vi "2P_AdapUprite_Linlin.vi"() -> ()   [LabVIEW 2015] (continued)
                    n2978 = Open VI Reference(type specifier VI Refnum (for type only)=refnum<vi> refnum, vi path=w6494, error in (no error)=w6492) -> (vi reference=w6490:refnum<vi>, error out=w6488:errorcluster)  [unwired: 3 in]
                    n2979 = call-by-ref "?"(reference=w6490, error in=w6488) -> (reference out=w6489:refnum<vi>, error out=w6487:errorcluster)  [unwired: 1 in]
                    n2980 = Close Reference(reference=w6489, error in (no error)=w6487) -> (error out=w6491:errorcluster)
                    n2981 = call <vilib>:"Unset Busy.vi"("error in (no error)"=w6491) -> ()  [unwired: 10 in, 1 out]
                    n2982 = local write "status"(w6491) -> ()
                  }
                  frame #2 {
                    n2983 = call "2pparameters.vi"("command"="get") -> ("params out"=w6521:T12)  [unwired: 1 in]
                    n2984 = Unbundle By Name(w6521) -> ("Xpixels Img"=w6520:i32, "Vx-min Img"=w6519:dbl, "VX-max Img"=w6518:dbl, "Ypixels Img"=w6517:i32, "Vy-min Img"=w6516:dbl, "Vy-max Img"=w6515:dbl, "Colormap"=w6514:u16, "square pixels"=w6513:bool, "square matrix"=w6512:bool, "Angle Img"=w6511:dbl, "Drawing Mode"=w6510:u16)
                    n2985 = local write "xpixels ref"(w6520) -> ()
                    n2986 = local write "Vx-min ref"(w6519) -> ()
                    n2987 = local write "Vx-max ref"(w6518) -> ()
                    n2988 = local write "ypixels ref"(w6517) -> ()
                    n2989 = local write "Vy-min ref"(w6516) -> ()
                    n2990 = local write "Vy-max ref"(w6515) -> ()
                    n2991 = local write "Colormap"(w6514) -> ()
                    n2992 = local write "Square pixels"(w6513) -> ()
                    n2993 = local write "square matrix"(w6512) -> ()
                    n2994 = local write "Angle ref"(w6511) -> ()
                    n2995 = local write "ROI Type"(w6510) -> ()
                    n2996 = call "2pparameters.vi"("command"="get") -> ("params out"=w6504:T12)  [unwired: 1 in]
                    n2997 = Unbundle By Name(w6504) -> ("Xpixels"=w6498:i32, "Vxminref"=w6502:dbl, "Vxmaxref"=w6501:dbl, "Ypixels"=w6497:i32, "Vyminref"=w6500:dbl, "Vymaxref"=w6499:dbl, "Colormap"=w6505:u16, "square pixels"=w6506:bool, "square matrix"=w6507:bool, "Angle draw"=w6508:dbl, "Drawing Mode"=w6509:u16)
                    n2998 = local write "Vy-max draw"(w6499) -> ()
                    n2999 = local write "Angle drawing"(w6508) -> ()
                    n3000 = local write "Colormap"(w6505) -> ()
                    n3001 = local write "Square pixels"(w6506) -> ()
                    n3002 = local write "square matrix"(w6507) -> ()
                    n3003 = local write "ROI Type"(w6509) -> ()
                    n3004 = local write "xpixels draw"(w6498) -> ()
                    n3005 = local write "ypixels draw"(w6497) -> ()
                    n3006 = local write "Vx-min draw"(w6502) -> ()
                    n3007 = local write "Vx-max draw"(w6501) -> ()
                    n3008 = local write "Vy-min draw"(w6500) -> ()
                  }
                  frame #3 {
                    n3009 = property on="ROI" class="Bool (strict)"("Val(Sgnl)"=FALSE ("x/y scan")) -> ()  [unwired: 2 in, 2 out]
                  }
                }
              }
            }
          }
          event "Xdattype": Value Change {
            n3010 = event-data() -> ()  [unwired: 1 in, 1 out]
            n3011 = case shown="True" "Xdattype" {
              frame False {
              }
              frame True {
                n3012 = stacked-sequence {
                  frame #0 {
                    n3013 = Current VI's Path() -> (path=w6534:path)
                    n3014 = Strip Path(path=w6534) -> (stripped path=w6535:path)  [unwired: 1 out]
                    n3015 = Build Path(base path=w6535, name or relative path="subVIs\\Misc\\Changedataconfig.vi") -> (appended path=w6533:path)
                    n3016 = call <vilib>:"Set Busy.vi"() -> ("error out"=w6531:errorcluster)  [unwired: 10 in, 1 out]
                    n3017 = Open VI Reference(type specifier VI Refnum (for type only)=refnum<vi> refnum, vi path=w6533, error in (no error)=w6531) -> (vi reference=w6526:refnum<vi>, error out=w6528:errorcluster)  [unwired: 3 in]
                    n3018 = call-by-ref "?"(reference=w6526, error in=w6528) -> (reference out=w6530:refnum<vi>, error out=w6529:errorcluster)  [unwired: 12 in]
                    n3019 = Close Reference(reference=w6530, error in (no error)=w6529) -> (error out=w6525:errorcluster)
                    "status" <- w6525
                    n3020 = call <vilib>:"Unset Busy.vi"("error in (no error)"=w6525) -> ()  [unwired: 10 in, 1 out]
                  }
                  frame #1 {
                    n3021 = property on="Xdattype" class="Bool (strict)"("Val(Sgnl)"=FALSE ("x/y scan")) -> ()  [unwired: 2 in, 2 out]
                  }
                }
              }
            }
          }
          event "XautoOD": Value Change {
            n3022 = event-data() -> ()  [unwired: 1 in, 1 out]
            n3023 = case shown="True" "XautoOD" {
              frame False {
              }
              frame True {
                n3024 = stacked-sequence {
                  frame #0 {
                    n3025 = Current VI's Path() -> (path=w6547:path)
                    n3026 = Strip Path(path=w6547) -> (stripped path=w6548:path)  [unwired: 1 out]
                    n3027 = Build Path(base path=w6548, name or relative path="subVIs\\Misc\\ChangeautoODs.vi") -> (appended path=w6546:path)
                    n3028 = call <vilib>:"Set Busy.vi"() -> ("error out"=w6544:errorcluster)  [unwired: 10 in, 1 out]
                    n3029 = Open VI Reference(type specifier VI Refnum (for type only)=refnum<vi> refnum, vi path=w6546, error in (no error)=w6544) -> (vi reference=w6539:refnum<vi>, error out=w6541:errorcluster)  [unwired: 3 in]
                    n3030 = call-by-ref "?"(reference=w6539, error in=w6541) -> (reference out=w6543:refnum<vi>, error out=w6542:errorcluster)  [unwired: 12 in]
                    n3031 = Close Reference(reference=w6543, error in (no error)=w6542) -> (error out=w6538:errorcluster)
                    "status 2" <- w6538
                    n3032 = call <vilib>:"Unset Busy.vi"("error in (no error)"=w6538) -> ()  [unwired: 10 in, 1 out]
                  }
                  frame #1 {
                    n3033 = property on="XautoOD" class="Bool (strict)"("Val(Sgnl)"=FALSE ("x/y scan")) -> ()  [unwired: 2 in, 2 out]
                  }
                }
              }
            }
          }
          event "SetMan": Value Change {
            n3034 = event-data() -> ()  [unwired: 1 in, 1 out]
            n3035 = case shown="True" "SetMan" {
              frame False {
              }
              frame True {
                n3036 = stacked-sequence {
                  frame #0 {
                    w6551 = u16 0 items=["Rectangle", "Circle", "Freeform Boundary", "Freeform Interior"] ("ROI Type")
                    n3037 = local write "ROI Type"(w6551) -> ()
                    n3038 = local read "Square pixels"() -> (w6557:bool)
                    n3039 = case shown="False" w6557 {
                      frame False {
                        n3040 = local read "square matrix"() -> (w6558:bool)
                        n3041 = case shown="False" w6558 {
                          frame False {
                            "ypixels ref" <- "ypixels"
                            "xpixels ref" <- "xpixels"
                          }
                          frame True {
                            n3042 = local read "xpixels"() -> (w6563:i32)
                            n3043 = local read "ypixels"() -> (w6562:i32)
                            n3044 = Max & Min(x=w6563, y=w6562) -> (max(x,y)=w6561:i32)  [unwired: 1 out]
                            n3045 = local write "xpixels ref"(w6561) -> ()
                            n3046 = local write "ypixels ref"(w6561) -> ()
                          }
                        }
                      }
                      frame True {
                        n3047 = local read "square matrix"() -> (w6564:bool)
                        n3048 = case shown="True" w6564 {
                          frame False {
                            n3049 = local read "Vxmax"() -> (w6578:dbl)
                            n3050 = local read "Vx-min"() -> (w6577:dbl)
                            n3051 = local read "Vy-max"() -> (w6573:dbl)
                            n3052 = local read "Vy-min"() -> (w6574:dbl)
                            n3053 = Subtract(x=w6573, y=w6574) -> (x-y=w6575:dbl)
                            n3054 = Subtract(x=w6578, y=w6577) -> (x-y=w6576:dbl)
                            n3055 = Absolute Value(x=w6575) -> (abs(x)=w6566:dbl)
                            n3056 = Absolute Value(x=w6576) -> (abs(x)=w6567:dbl)
                            n3057 = Divide(x=w6567, y=w6566) -> (x/y=w6572:dbl)
                            n3058 = Greater Or Equal?(x=w6567, y=w6566) -> (x >= y?=w6565:bool)
                            n3059 = local read "xpixels"() -> (w6571:i32)
                            n3060 = local read "ypixels"() -> (w6568:i32)
                            n3061 = case shown="False" w6565 {
                              tunnel: w6572 -> [w6583 w6586]
                              tunnel: w6571 -> [w6580 _]
                              tunnel: [w6580 w6585] -> w6570
                              tunnel: [w6579 w6584] -> w6569
                              tunnel: w6568 -> [_ w6584]
                              frame False {
                                n3062 = To Double Precision Float(number=w6580) -> (double precision float=w6582:dbl)
                                n3063 = Divide(x=w6582, y=w6583) -> (x/y=w6581:dbl)
                                n3064 = To Long Integer(number=w6581) -> (32bit integer=w6579:i32)
                              }
                              frame True {
                                n3065 = To Double Precision Float(number=w6584) -> (double precision float=w6588:dbl)
                                n3066 = Multiply(x=w6588, y=w6586) -> (x*y=w6587:dbl)
                                n3067 = To Long Integer(number=w6587) -> (32bit integer=w6585:i32)
                              }
                            }
                            n3068 = local write "ypixels ref"(w6569) -> ()
                            n3069 = local write "xpixels ref"(w6570) -> ()
                          }
                          frame True {
                          }
                        }
                      }
                    }
                    "Vx-max ref" <- "Vxmax"
                    "Vx-min ref" <- "Vx-min"
                    "Vy-max ref" <- "Vy-max"
                    "Vy-min ref" <- "Vy-min"
                    "Angle ref" <- "Angle"
                  }
                  frame #1 {
                    n3070 = property on="SetMan" class="Bool (strict)"("Val(Sgnl)"=FALSE ("Value (Signaling)")) -> ()  [unwired: 2 in, 2 out]
                  }
                }
              }
            }
          }
          event "QuickSetMan": Value Change {
            n3071 = event-data() -> ()  [unwired: 1 in, 6 out]
            n3072 = case shown="True" "QuickSetMan" {
              tunnel: "Vpp" -> [_ w6594]
              tunnel: "px" -> [_ w6593]
              frame False {
              }
              frame True {
                n3073 = stacked-sequence {
                  tunnel: w6594 -> [w6599 _]
                  tunnel: w6593 -> [w6595 _]
                  frame #0 {
                    w6601 = u16 0 items=["Rectangle", "Circle", "Freeform Boundary", "Freeform Interior"] ("ROI Type")
                    n3074 = Divide(x=w6599, y=2.0) -> (x/y=w6598:dbl)
                    n3075 = Negate(x=w6598) -> (-x=w6597:dbl)
                    n3076 = local write "ROI Type"(w6601) -> ()
                    n3077 = local write "Vx-min ref"(w6597) -> ()
                    n3078 = local write "Vy-max ref"(w6598) -> ()
                    n3079 = local write "Vx-max ref"(w6598) -> ()
                    n3080 = local write "Vy-min ref"(w6597) -> ()
                    n3081 = local write "Angle ref"(0.0 ("Angle ref 2")) -> ()
                    n3082 = local write "xpixels ref"(w6595) -> ()
                    n3083 = local write "ypixels ref"(w6595) -> ()
                  }
                  frame #1 {
                    n3084 = property on="QuickSetMan" class="Bool (strict)"("Val(Sgnl)"=FALSE ("Value (Signaling)")) -> ()  [unwired: 2 in, 2 out]
                  }
                }
              }
            }
          }
          event "SetMan 2": Value Change {
            n3085 = event-data() -> ()  [unwired: 1 in, 1 out]
            n3086 = case shown="True" "SetMan 2" {
              frame False {
              }
              frame True {
                n3087 = stacked-sequence {
                  frame #0 {
                    n3088 = local write "Vx-ref"("Vx") -> ()
                    n3089 = local write "Vy-ref"("Vy") -> ()
                  }
                  frame #1 {
                    n3090 = property on="SetMan 2" class="Bool (strict)"("Val(Sgnl)"=FALSE ("Value (Signaling)")) -> ()  [unwired: 2 in, 2 out]
                  }
                }
              }
            }
          }
          event "Reset Coords": Value Change {
            n3091 = event-data() -> ("NewVal"=w6607:bool)  [unwired: 1 in, 5 out]
            n3092 = case shown="True" w6607 {
              frame False {
              }
              frame True {
                n3093 = stacked-sequence {
                  frame #0 {
                    n3094 = local write "xpixels"(256 ("xpixels")) -> ()
                    n3095 = local write "ypixels"(256 ("ypixels")) -> ()
                    n3096 = local write "Vxmax"(9.0 ("Vx-max")) -> ()
                    n3097 = local write "Vx-min"(-9.0 ("Vx-min")) -> ()
                    n3098 = local write "Vy-max"(9.0 ("Vy-max")) -> ()
                    n3099 = local write "Vy-min"(-9.0 ("Vy-min")) -> ()
                    n3100 = local write "Angle"(0.0 ("Angle")) -> ()
                  }
                  frame #1 {
                    n3101 = property on="Reset Coords" class="Bool (strict)"("Value"=FALSE ("TROI")) -> ()  [unwired: 2 in, 2 out]
                  }
                }
              }
            }
          }
          event "TROI": Value Change {
            n3102 = event-data() -> ()  [unwired: 1 in, 1 out]
            n3103 = case shown="True" "TROI" {
              frame False {
              }
              frame True {
                n3104 = stacked-sequence {
                  frame #0 {
                    n3105 = local read "Vy-min ref"() -> (w6621:dbl)
                    n3106 = local read "Vy-max ref"() -> (w6620:dbl)
                    n3107 = local read "Vx-max ref"() -> (w6618:dbl)
                    n3108 = local read "Vx-min ref"() -> (w6619:dbl)
                    n3109 = local read "ypixels ref"() -> (w6623:i32)
                    n3110 = local read "xpixels ref"() -> (w6622:i32)
                    n3111 = local read "Angle ref"() -> (w6617:dbl)
                    n3112 = local write "Angle"(w6617) -> ()
                    n3113 = local write "xpixels"(w6622) -> ()
                    n3114 = local write "Vy-min"(w6621) -> ()
                    n3115 = local write "Vy-max"(w6620) -> ()
                    n3116 = local write "Vx-min"(w6619) -> ()
                    n3117 = local write "ypixels"(w6623) -> ()
                    n3118 = local write "Vxmax"(w6618) -> ()
                  }
                  frame #1 {
                    n3119 = property on="TROI" class="Bool (strict)"("Value"=FALSE ("TROI")) -> ()  [unwired: 2 in, 2 out]
                  }
                }
              }
            }
          }
          event "TROI 2": Value Change {
            n3120 = event-data() -> ()  [unwired: 1 in, 1 out]
            n3121 = case shown="True" "TROI 2" {
              frame False {
              }
              frame True {
                n3122 = stacked-sequence {
                  frame #0 {
                    n3123 = local read "Vx-ref"() -> (w6626:dbl)
                    n3124 = local read "Vy-ref"() -> (w6627:dbl)
                    n3125 = local write "Vx"(w6626) -> ()
                    n3126 = local write "Vy"(w6627) -> ()
                  }
                  frame #1 {
                    n3127 = property on="TROI 2" class="Bool (strict)"("Value"=FALSE ("TROI")) -> ()  [unwired: 2 in, 2 out]
                  }
                }
              }
            }
          }
          event "Square pixels": Value Change {
            n3128 = event-data() -> ()  [unwired: 1 in, 1 out]
            n3129 = case shown="True" "Square pixels" {
              frame False {
              }
              frame True {
                n3130 = property on="square matrix" class="Bool (strict)"("Value"=FALSE ("square matrix")) -> ()  [unwired: 2 in, 2 out]
                n3131 = property on="Square pixels" class="Bool (strict)"("Value"=TRUE ("square matrix")) -> ()  [unwired: 2 in, 2 out]
              }
            }
          }
          event "square matrix": Value Change {
            n3132 = event-data() -> ()  [unwired: 1 in, 1 out]
            n3133 = case shown="True" "square matrix" {
              frame False {
              }
              frame True {
                n3134 = property on="square matrix" class="Bool (strict)"("Value"=TRUE ("square matrix")) -> ()  [unwired: 2 in, 2 out]
                n3135 = property on="Square pixels" class="Bool (strict)"("Value"=FALSE ("square matrix")) -> ()  [unwired: 2 in, 2 out]
              }
            }
          }
          event "up", "downright", "down", "downleft", "right", "left", "upright", "upleft": Value Change {
            n3136 = event-data() -> ()  [unwired: 1 in, 6 out]
            n3137 = local read "downright"() -> (w6640:bool)
            n3138 = local read "downleft"() -> (w6642:bool)
            n3139 = local read "upright"() -> (w6638:bool)
            n3140 = local read "upleft"() -> (w6636:bool)
            n3141 = local read "down"() -> (w6641:bool)
            n3142 = local read "right"() -> (w6639:bool)
            n3143 = local read "left"() -> (w6643:bool)
            n3144 = local read "up"() -> (w6637:bool)
            n3145 = Compound Arithmetic op=OR(w6636, w6637, w6638, w6639, w6640, w6641, w6642, w6643) -> (w6635:bool)
            n3146 = case shown="True" w6635 {
              frame False {
              }
              frame True {
                n3147 = stacked-sequence {
                  frame #0 {
                    n3148 = local read "downright"() -> (w6645:bool)
                    n3149 = local read "downleft"() -> (w6647:bool)
                    n3150 = local read "BigSmall"() -> (w6644:bool)
                    n3151 = local read "upright"() -> (w6649:bool)
                    n3152 = local read "upleft"() -> (w6652:bool)
                    n3153 = local read "down"() -> (w6648:bool)
                    n3154 = local read "right"() -> (w6650:bool)
                    n3155 = local read "left"() -> (w6646:bool)
                    n3156 = local read "up"() -> (w6651:bool)
                    n3157 = call "movestageparams.vi"("command"="get") -> ("Params out"=w6655:T23)  [unwired: 1 in]
                    n3158 = Bundle By Name(cluster=w6655, "upleft"=w6652, "up"=w6651, "upright"=w6649, "right"=w6650, "downright"=w6645, "down"=w6648, "downleft"=w6647, "left"=w6646, "Bigsmall"=w6644) -> (w6656:T23)
                    n3159 = call "movestageparams.vi"("Params in"=w6656, "command"="set") -> ()  [unwired: 1 out]
                  }
                  frame #1 {
                  }
                  frame #2 {
                    n3160 = call "movestage.vi"() -> ()  [unwired: 12 in]
                  }
                  frame #3 {
                    w6657 = FALSE ("OK Button")
                    w6658 = FALSE ("OK Button")
                    n3161 = property on="down" class="Bool (strict)"("Value"=w6658) -> ()  [unwired: 2 in, 2 out]
                    n3162 = property on="up" class="Bool (strict)"("Value"=w6658) -> ()  [unwired: 2 in, 2 out]
                    n3163 = property on="right" class="Bool (strict)"("Value"=w6658) -> ()  [unwired: 2 in, 2 out]
                    n3164 = property on="left" class="Bool (strict)"("Value"=w6658) -> ()  [unwired: 2 in, 2 out]
                    n3165 = property on="upright" class="Bool (strict)"("Value"=w6657) -> ()  [unwired: 2 in, 2 out]
                    n3166 = property on="downleft" class="Bool (strict)"("Value"=w6657) -> ()  [unwired: 2 in, 2 out]
                    n3167 = property on="downright" class="Bool (strict)"("Value"=w6657) -> ()  [unwired: 2 in, 2 out]
                    n3168 = property on="upleft" class="Bool (strict)"("Value"=w6657) -> ()  [unwired: 2 in, 2 out]
                  }
                }
              }
            }
          }
          event "finite samples": Value Change {
            n3169 = event-data() -> ("NewVal"=w6659:bool)  [unwired: 1 in]
            n3170 = flat-sequence {
              tunnel: w6659 -> [w6660]
              frame #0 {
                n3171 = case shown="True" w6660 {
                  frame False {
                    w6661 = FALSE ("wavdet")
                    n3172 = property on="continuous" class="Bool (strict)"("Value"=TRUE ("continuous for display")) -> ()  [unwired: 2 in, 2 out]
                    n3173 = property on="wavdet" class="Bool (strict)"("Value"=w6661) -> ()  [unwired: 2 in, 2 out]
                    n3174 = property on="save\ndata" class="Bool (strict)"("Value"=w6661) -> ()  [unwired: 2 in, 2 out]
                    n3175 = property on="# of frames" class="DigNum (strict)"("DisabledEnum"=T7."Disabled and Grayed Out" ("Disabled")) -> ()  [unwired: 2 in, 2 out]
                    n3176 = property on="save\ndata" class="Bool (strict)"("DisabledEnum"=T7."Disabled and Grayed Out" ("Disabled")) -> ()  [unwired: 2 in, 2 out]
                    "Save tab" <- enum32{"withsave", "withoutsave"}."withsave" ("Save tab")
                  }
                  frame True {
                    w6668 = FALSE ("continuous for display")
                    n3177 = property on="continuous" class="Bool (strict)"("Value"=w6668) -> ()  [unwired: 2 in, 2 out]
                    n3178 = property on="wavdet" class="Bool (strict)"("Value"=w6668) -> ()  [unwired: 2 in, 2 out]
                    n3179 = local write "Save tab"(enum32{"withsave", "withoutsave"}."withsave" ("Save tab")) -> ()
                    n3180 = property on="save\ndata" class="Bool (strict)"("DisabledEnum"=T7."Enabled" ("Disabled")) -> ()  [unwired: 2 in, 2 out]
                    n3181 = property on="save\ndata" class="Bool (strict)"("Value"=TRUE ("save\ndata")) -> ()  [unwired: 2 in, 2 out]
                    n3182 = property on="# of frames" class="DigNum (strict)"("DisabledEnum"=T7."Enabled" ("Disabled")) -> ()  [unwired: 2 in, 2 out]
                  }
                }
              }
              frame #1 {
                n3183 = local read "finite samples"() -> (w6677:bool)
                n3184 = local read "continuous"() -> (w6676:bool)
                n3185 = local read "wavdet"() -> (w6675:bool)
                n3186 = call "2pparameters.vi"("command"="get") -> ("params out"=w6671:T12)  [unwired: 1 in]
                n3187 = Bundle By Name(cluster=w6671, "finite"=w6677, "cont"=w6676, "wavdet"=w6675) -> (w6674:T12)
                n3188 = call "2pparameters.vi"("Params in"=w6674, "command"="set") -> ()  [unwired: 1 out]
              }
            }
          }
          event "continuous": Value Change {
            n3189 = event-data() -> ("NewVal"=w6678:bool)  [unwired: 1 in]
            n3190 = flat-sequence {
              tunnel: w6678 -> [w6679]
              frame #0 {
                n3191 = case shown="True" w6679 {
                  frame False {
                    n3192 = property on="finite samples" class="Bool (strict)"("Value"=TRUE ("finite samples for recording")) -> ()  [unwired: 2 in, 2 out]
                    n3193 = property on="save\ndata" class="Bool (strict)"("Value"=TRUE ("save\ndata")) -> ()  [unwired: 2 in, 2 out]
                    n3194 = property on="wavdet" class="Bool (strict)"("Value"=FALSE ("wavdet")) -> ()  [unwired: 2 in, 2 out]
                    n3195 = local write "Save tab"(enum32{"withsave", "withoutsave"}."withsave" ("Save tab")) -> ()
                    n3196 = property on="# of frames" class="DigNum (strict)"("DisabledEnum"=T7."Enabled" ("Disabled")) -> ()  [unwired: 2 in, 2 out]
                    n3197 = property on="save\ndata" class="Bool (strict)"("DisabledEnum"=T7."Enabled" ("Disabled")) -> ()  [unwired: 2 in, 2 out]
                  }
                  frame True {
                    w6686 = FALSE ("finite samples for recording")
                    n3198 = property on="finite samples" class="Bool (strict)"("Value"=w6686) -> ()  [unwired: 2 in, 2 out]
                    n3199 = property on="wavdet" class="Bool (strict)"("Value"=w6686) -> ()  [unwired: 2 in, 2 out]
                    n3200 = property on="save\ndata" class="Bool (strict)"("Value"=w6686) -> ()  [unwired: 2 in, 2 out]
                    n3201 = local write "Save tab"(enum32{"withsave", "withoutsave"}."withsave" ("Save tab")) -> ()
                    n3202 = property on="# of frames" class="DigNum (strict)"("DisabledEnum"=T7."Disabled and Grayed Out" ("Disabled")) -> ()  [unwired: 2 in, 2 out]
                    n3203 = property on="save\ndata" class="Bool (strict)"("DisabledEnum"=T7."Disabled and Grayed Out" ("Disabled")) -> ()  [unwired: 2 in, 2 out]
                  }
                }
              }
              frame #1 {
                n3204 = local read "finite samples"() -> (w6696:bool)
                n3205 = local read "continuous"() -> (w6695:bool)
                n3206 = local read "wavdet"() -> (w6694:bool)
                n3207 = call "2pparameters.vi"("command"="get") -> ("params out"=w6690:T12)  [unwired: 1 in]
                n3208 = Bundle By Name(cluster=w6690, "finite"=w6696, "cont"=w6695, "wavdet"=w6694) -> (w6693:T12)
                n3209 = call "2pparameters.vi"("Params in"=w6693, "command"="set") -> ()  [unwired: 1 out]
              }
            }
          }
          event "wavdet": Value Change {
            n3210 = event-data() -> ("NewVal"=w6697:bool)  [unwired: 1 in]
            n3211 = flat-sequence {
              tunnel: w6697 -> [w6698]
              frame #0 {
                n3212 = case shown="False" w6698 {
                  frame False {
                    n3213 = property on="finite samples" class="Bool (strict)"("Value"=TRUE ("finite samples for recording")) -> ()  [unwired: 2 in, 2 out]
                    n3214 = property on="continuous" class="Bool (strict)"("Value"=FALSE ("continuous")) -> ()  [unwired: 2 in, 2 out]
                    n3215 = local write "Save tab"(enum32{"withsave", "withoutsave"}."withsave" ("Save tab")) -> ()
                    n3216 = property on="save\ndata" class="Bool (strict)"("DisabledEnum"=T7."Enabled" ("Disabled")) -> ()  [unwired: 2 in, 2 out]
                    n3217 = property on="# of frames" class="DigNum (strict)"("DisabledEnum"=T7."Enabled" ("Disabled")) -> ()  [unwired: 2 in, 2 out]
                    n3218 = property on="save\ndata" class="Bool (strict)"("Value"=TRUE ("save\ndata")) -> ()  [unwired: 2 in, 2 out]
                  }
                  frame True {
                    w6707 = FALSE ("finite samples for recording")
                    n3219 = property on="finite samples" class="Bool (strict)"("Value"=w6707) -> ()  [unwired: 2 in, 2 out]
                    n3220 = property on="continuous" class="Bool (strict)"("Value"=w6707) -> ()  [unwired: 2 in, 2 out]
                    n3221 = property on="save\ndata" class="Bool (strict)"("DisabledEnum"=T7."Enabled" ("Disabled")) -> ()  [unwired: 2 in, 2 out]
                    n3222 = local write "Save tab"(enum32{"withsave", "withoutsave"}."withsave" ("Save tab")) -> ()
                    n3223 = property on="# of frames" class="DigNum (strict)"("DisabledEnum"=T7."Disabled" ("Disabled")) -> ()  [unwired: 2 in, 2 out]
                    n3224 = property on="save\ndata" class="Bool (strict)"("Value"=TRUE ("save\ndata")) -> ()  [unwired: 2 in, 2 out]
                  }
                }
              }
              frame #1 {
                n3225 = local read "finite samples"() -> (w6710:bool)
                n3226 = local read "continuous"() -> (w6711:bool)
                n3227 = local read "wavdet"() -> (w6712:bool)
                n3228 = call "2pparameters.vi"("command"="get") -> ("params out"=w6716:T12)  [unwired: 1 in]
                n3229 = Bundle By Name(cluster=w6716, "finite"=w6710, "cont"=w6711, "wavdet"=w6712) -> (w6713:T12)
                n3230 = call "2pparameters.vi"("Params in"=w6713, "command"="set") -> ()  [unwired: 1 out]
              }
            }
          }
          event "cursors": Value Change {
            n3231 = event-data() -> ()  [unwired: 1 in, 5 out]
            n3232 = case shown="True" "cursors" {
              frame False {
                n3233 = property on="img_CH1" class="IntGraph (strict)"("Active Cursor"=u32 0, "Cursor.Cursor Style"=u8 0 ("Cursor Style"), "Cursor.Cursor Point Style"=u8 0 ("Cursor Point Style")) -> ("Cursor.Cursor Position:Cursor X"=w6721:dbl, "Cursor.Cursor Position:Cursor Y"=w6722:dbl)  [unwired: 2 in, 2 out]
                n3234 = property on="img_CH2" class="IntGraph (strict)"("Active Cursor"=u32 0, "Cursor.Cursor Style"=u8 0 ("Cursor Style"), "Cursor.Cursor Point Style"=u8 0 ("Cursor Point Style")) -> ()  [unwired: 2 in, 2 out]
                n3235 = local write "cursor x [pixel]"(w6721) -> ()
                n3236 = local write "cursor y [pixel]"(w6722) -> ()
              }
              frame True {
                n3237 = stacked-sequence {
                  frame #0 {
                    n3238 = call "2pparameters.vi"("command"="get") -> ("params out"=w6737:T12)  [unwired: 1 in]
                    n3239 = Unbundle By Name(w6737) -> ("Xpixels Img"=w6738:i32, "Ypixels Img"=w6735:i32)
                    n3240 = To Double Precision Float(number=w6735) -> (double precision float=w6729:dbl)
                    n3241 = To Double Precision Float(number=w6738) -> (double precision float=w6734:dbl)
                    n3242 = Divide(x=w6729, y=2.0) -> (x/y=w6730:dbl)
                    n3243 = Divide(x=w6734, y=2.0) -> (x/y=w6732:dbl)
                    n3244 = Round To Nearest(number=w6730) -> (nearest integer value=w6728:dbl)
                    n3245 = Round To Nearest(number=w6732) -> (nearest integer value=w6731:dbl)
                    n3246 = property on="img_CH1" class="IntGraph (strict)"("Active Cursor"=u32 0, "Cursor.Cursor Style"=u8 8 ("Cursor Style"), "Cursor.Cursor Point Style"=u8 5 ("Cursor Point Style"), "Cursor.Cursor Position:Cursor X"=w6731, "Cursor.Cursor Position:Cursor Y"=w6728, "Cursor.Visible"=TRUE) -> ()  [unwired: 2 in, 2 out]
                  }
                  frame #1 {
                    n3247 = call "2pparameters.vi"("command"="get") -> ("params out"=w6757:T12)  [unwired: 1 in]
                    n3248 = call "2pparameters.vi"("command"="get") -> ("params out"=w6755:T12)  [unwired: 1 in]
                    n3249 = property on="img_CH1" class="IntGraph (strict)"("Active Cursor"=u32 0, "Cursor.Cursor Style"=u8 8 ("Cursor Style"), "Cursor.Cursor Point Style"=u8 5 ("Cursor Point Style")) -> ("Cursor.Cursor Position:Cursor X"=w6750:dbl, "Cursor.Cursor Position:Cursor Y"=w6749:dbl, "Cursor.Cursor Index"=w6772:i32, "Cursor.Cursor Plot"=w6771:i32, "Cursor.Visible"=w6742:bool)  [unwired: 2 in, 2 out]
                    "cursor x [pixel]" <- w6750
                    "cursor y [pixel]" <- w6749
                    n3250 = Unbundle By Name(w6757) -> ("Vy-max Img"=w6759:dbl, "Vy-min Img"=w6746:dbl, "Ypixels Img"=w6761:i32)
                    n3251 = Unbundle By Name(w6755) -> ("VX-max Img"=w6756:dbl, "Vx-min Img"=w6744:dbl, "Xpixels Img"=w6760:i32)
                    n3252 = Subtract(x=w6759, y=w6746) -> (x-y=w6764:dbl)
                    n3253 = Subtract(x=w6756, y=w6744) -> (x-y=w6762:dbl)
                    n3254 = local read "img_CH2"() -> (w6768:sgl[][])
                    n3255 = To Double Precision Float(number=w6760) -> (double precision float=w6763:dbl)
                    n3256 = local read "img_CH1"() -> (w6769:sgl[][])
                    n3257 = To Double Precision Float(number=w6761) -> (double precision float=w6765:dbl)
                    n3258 = Index Array(array=w6769, index (row)=w6772, index (col)=w6771) -> (element=→"value CH 1":sgl)
                    n3259 = Index Array(array=w6768, index (row)=w6772, index (col)=w6771) -> (element=→"value CH 2":sgl)
                    n3260 = Divide(x=w6762, y=w6763) -> (x/y=w6766:dbl)
                    n3261 = Divide(x=w6764, y=w6765) -> (x/y=w6767:dbl)
                    n3262 = Multiply(x=w6750, y=w6766) -> (x*y=w6745:dbl)
                    n3263 = Multiply(x=w6749, y=w6767) -> (x*y=w6748:dbl)
                    n3264 = property on="img_CH2" class="IntGraph (strict)"("Active Cursor"=u32 0, "Cursor.Cursor Style"=u8 8 ("Cursor Style"), "Cursor.Cursor Point Style"=u8 5 ("Cursor Point Style"), "Cursor.Cursor Position:Cursor X"=w6750, "Cursor.Cursor Position:Cursor Y"=w6749, "Cursor.Visible"=w6742) -> ()  [unwired: 2 in, 2 out]
                    n3265 = Add(x=w6745, y=w6744) -> (x+y=w6743:dbl)
                    n3266 = Add(x=w6748, y=w6746) -> (x+y=w6747:dbl)
                    n3267 = local write "Vx-ref"(w6743) -> ()
                    n3268 = local write "Vy-ref"(w6747) -> ()
                  }
                }
              }
            }
          }
          event "img_CH1": Cursor Move {
            n3269 = event-data() -> ("CursIdx"=w6777:i32)  [unwired: 1 in]
            n3270 = Equal To 0?(x=w6777) -> (x = 0?=w6778:bool)
            n3271 = case shown="True" w6778 {
              frame False {
              }
              frame True {
                n3272 = call "2pparameters.vi"("command"="get") -> ("params out"=w6798:T12)  [unwired: 1 in]
                n3273 = call "2pparameters.vi"("command"="get") -> ("params out"=w6800:T12)  [unwired: 1 in]
                n3274 = property on="img_CH1" class="IntGraph (strict)"("Active Cursor"=u32 0, "Cursor.Cursor Style"=u8 8 ("Cursor Style"), "Cursor.Cursor Point Style"=u8 5 ("Cursor Point Style")) -> ("Cursor.Cursor Position:Cursor X"=w6787:dbl, "Cursor.Cursor Position:Cursor Y"=w6786:dbl, "Cursor.Cursor Plot"=w6806:i32, "Cursor.Cursor Index"=w6805:i32, "Cursor.Visible"=w6779:bool)  [unwired: 2 in, 2 out]
                n3275 = Unbundle By Name(w6798) -> ("Vy-max Img"=w6796:dbl, "Vy-min Img"=w6785:dbl, "Ypixels Img"=w6794:i32)
                n3276 = Unbundle By Name(w6800) -> ("VX-max Img"=w6799:dbl, "Vx-min Img"=w6780:dbl, "Xpixels Img"=w6795:i32)
                n3277 = Subtract(x=w6796, y=w6785) -> (x-y=w6791:dbl)
                n3278 = Subtract(x=w6799, y=w6780) -> (x-y=w6793:dbl)
                n3279 = local write "cursor x [pixel]"(w6787) -> ()
                n3280 = local write "cursor y [pixel]"(w6786) -> ()
                n3281 = To Double Precision Float(number=w6795) -> (double precision float=w6792:dbl)
                n3282 = To Double Precision Float(number=w6794) -> (double precision float=w6790:dbl)
                n3283 = local read "img_CH2"() -> (w6807:sgl[][])
                n3284 = local read "img_CH1"() -> (w6810:sgl[][])
                n3285 = Index Array(array=w6807, index (row)=w6806, index (col)=w6805) -> (element=w6808:sgl)
                n3286 = Index Array(array=w6810, index (row)=w6806, index (col)=w6805) -> (element=w6809:sgl)
                n3287 = Divide(x=w6793, y=w6792) -> (x/y=w6789:dbl)
                n3288 = Divide(x=w6791, y=w6790) -> (x/y=w6788:dbl)
                n3289 = local write "value CH 2"(w6808) -> ()
                n3290 = Multiply(x=w6787, y=w6789) -> (x*y=w6782:dbl)
                n3291 = local write "value CH 1"(w6809) -> ()
                n3292 = Multiply(x=w6786, y=w6788) -> (x*y=w6784:dbl)
                n3293 = Add(x=w6782, y=w6780) -> (x+y=w6781:dbl)
                n3294 = local write "Vx-ref"(w6781) -> ()
                n3295 = Add(x=w6784, y=w6785) -> (x+y=w6783:dbl)
                n3296 = property on="img_CH2" class="IntGraph (strict)"("Active Cursor"=u32 0, "Cursor.Cursor Style"=u8 8 ("Cursor Style"), "Cursor.Cursor Point Style"=u8 5 ("Cursor Point Style"), "Cursor.Cursor Position:Cursor X"=w6787, "Cursor.Cursor Position:Cursor Y"=w6786, "Cursor.Visible"=w6779) -> ()  [unwired: 2 in, 2 out]
                n3297 = local write "Vy-ref"(w6783) -> ()
              }
            }
          }
          event "img_CH2": Cursor Move {
            n3298 = event-data() -> ("CursIdx"=w6814:i32)  [unwired: 1 in]
            n3299 = Equal To 0?(x=w6814) -> (x = 0?=w6815:bool)
            n3300 = case shown="True" w6815 {
              frame False {
              }
              frame True {
                n3301 = property on="img_CH2" class="IntGraph (strict)"("Active Cursor"=u32 0, "Cursor.Cursor Style"=u8 8 ("Cursor Style"), "Cursor.Cursor Point Style"=u8 5 ("Cursor Point Style")) -> ("Cursor.Cursor Position:Cursor X"=w6823:dbl, "Cursor.Cursor Position:Cursor Y"=w6824:dbl, "Cursor.Cursor Plot"=w6843:i32, "Cursor.Cursor Index"=w6842:i32, "Cursor.Visible"=w6816:bool)  [unwired: 2 in, 2 out]
                n3302 = call "2pparameters.vi"("command"="get") -> ("params out"=w6835:T12)  [unwired: 1 in]
                n3303 = call "2pparameters.vi"("command"="get") -> ("params out"=w6837:T12)  [unwired: 1 in]
                n3304 = local read "img_CH1"() -> (w6847:sgl[][])
                n3305 = local read "img_CH2"() -> (w6844:sgl[][])
                n3306 = local write "cursor x [pixel]"(w6823) -> ()
                n3307 = local write "cursor y [pixel]"(w6824) -> ()
                n3308 = Unbundle By Name(w6835) -> ("Vy-max Img"=w6833:dbl, "Vy-min Img"=w6818:dbl, "Ypixels Img"=w6831:i32)
                n3309 = Unbundle By Name(w6837) -> ("VX-max Img"=w6836:dbl, "Vx-min Img"=w6821:dbl, "Xpixels Img"=w6832:i32)
                n3310 = Index Array(array=w6847, index (row)=w6843, index (col)=w6842) -> (element=w6846:sgl)
                n3311 = Index Array(array=w6844, index (row)=w6843, index (col)=w6842) -> (element=w6845:sgl)
                n3312 = local write "value CH 2"(w6845) -> ()
                n3313 = local write "value CH 1"(w6846) -> ()
                n3314 = Subtract(x=w6833, y=w6818) -> (x-y=w6828:dbl)
                n3315 = Subtract(x=w6836, y=w6821) -> (x-y=w6830:dbl)
                n3316 = To Double Precision Float(number=w6832) -> (double precision float=w6829:dbl)
                n3317 = To Double Precision Float(number=w6831) -> (double precision float=w6827:dbl)
                n3318 = Divide(x=w6830, y=w6829) -> (x/y=w6826:dbl)
                n3319 = Divide(x=w6828, y=w6827) -> (x/y=w6825:dbl)
                n3320 = Multiply(x=w6823, y=w6826) -> (x*y=w6822:dbl)
                n3321 = Multiply(x=w6824, y=w6825) -> (x*y=w6819:dbl)
                n3322 = property on="img_CH1" class="IntGraph (strict)"("Active Cursor"=u32 0, "Cursor.Cursor Style"=u8 8 ("Cursor Style"), "Cursor.Cursor Point Style"=u8 5 ("Cursor Point Style"), "Cursor.Cursor Position:Cursor X"=w6823, "Cursor.Cursor Position:Cursor Y"=w6824, "Cursor.Visible"=w6816) -> ()  [unwired: 2 in, 2 out]
                n3323 = Add(x=w6822, y=w6821) -> (x+y=→"Vx-ref":dbl)
                n3324 = Add(x=w6819, y=w6818) -> (x+y=→"Vy-ref":dbl)
              }
            }
          }
          event "Focus": Value Change {
            n3325 = event-data() -> ()  [unwired: 1 in, 6 out]
            n3326 = flat-sequence {
              frame #0 {
                n3327 = local read "Focus"() -> (w6851:bool)
                n3328 = case shown="True" w6851 {
                  frame False {
                  }
                  frame True {
                    n3329 = local read "Vx-ref"() -> (w6855:dbl)
                    n3330 = local read "Vy-ref"() -> (w6854:dbl)
                    n3331 = local read "zV"() -> (w6852:dbl)
                    n3332 = call "focusvi.vi"("zc"=w6852, "yc"=w6854, "xc"=w6855) -> ("finalz"=→"zV":dbl)
                  }
                }
              }
              frame #1 {
                n3333 = local write "Focus"(FALSE ("Focus")) -> ()
              }
            }
          }
          event "auto shutter": Value Change {
            n3334 = event-data() -> ()  [unwired: 1 in, 6 out]
            n3335 = call "2pparameters.vi"("command"="get") -> ("params out"=w6859:T12)  [unwired: 1 in]
            n3336 = in-place {
              n3337 = in-place-cluster #45(w6859) -> ()  [unwired: 1 out]
              n3338 = local read "auto shutter"() -> (w6861:bool)
              n3339 = in-place-cluster #45("autoshutter"=w6861) -> (w6857:T12)
            }
            n3340 = call "2pparameters.vi"("Params in"=w6857, "command"="set") -> ()  [unwired: 1 out]
          }
          event "auto OD": Value Change {
            n3341 = event-data() -> ()  [unwired: 1 in, 6 out]
            n3342 = call "2pparameters.vi"("command"="get") -> ("params out"=w6864:T12)  [unwired: 1 in]
            n3343 = in-place {
              n3344 = in-place-cluster #46(w6864) -> ()  [unwired: 1 out]
              n3345 = local read "auto OD"() -> (w6866:bool)
              n3346 = in-place-cluster #46("auto OD"=w6866) -> (w6862:T12)
            }
            n3347 = call "2pparameters.vi"("Params in"=w6862, "command"="set") -> ()  [unwired: 1 out]
          }
          event "ODfilt": Value Change {
            n3348 = event-data() -> ("OldVal"=w6869:u16)  [unwired: 1 in, 5 out]
            n3349 = call "2pparameters.vi"("command"="get") -> ("params out"=w6867:T12)  [unwired: 1 in]
            n3350 = local read "ODfilt"() -> (w6870:u16)
            n3351 = call "filterwheelcontrol_nothorlabslib.vi"("Current OD filt"=w6869, "New ODfilt"=w6870) -> ()  [unwired: 1 in]
            n3352 = in-place {
              in-place-border: w6870 -> [w6873]
              n3353 = in-place-cluster #47(w6867) -> ()  [unwired: 1 out]
              n3354 = in-place-cluster #47("ODfilt"=w6873) -> (w6871:T12)
            }
            n3355 = call "2pparameters.vi"("Params in"=w6871, "command"="set") -> ()  [unwired: 1 out]
          }
          event "Use external 100KHz Clock": Value Change {
            n3356 = event-data() -> ("NewVal"=w6875:bool)  [unwired: 1 in, 5 out]
            n3357 = control-ref of="Measurement"() -> (w6877:refnum<vi>)
            n3358 = property class="Enum (strict)"(reference=w6877) -> ("Value"=w6876:T4)  [unwired: 1 in, 2 out]
            n3359 = case shown="\"Timetrace\"" w6876 {
              tunnel: [w6893 w6894] -> w6874
              frame "X-Y-t movie", "X-Y-Z stack", Default {
                n3360 = control-ref of="Sampling rate"() -> (w6893:refnum<vi>)
              }
              frame "Timetrace" {
                n3361 = control-ref of="srateAODOtt"() -> (w6894:refnum<vi>)
              }
            }
            n3362 = case shown="False" w6875 {
              tunnel: w6874 -> [w6878 w6885]
              frame False {
                n3363 = call "2pparameters.vi"("command"="get") -> ("params out"=w6882:T12)  [unwired: 1 in]
                n3364 = Bundle By Name(cluster=w6882, "External 100KHz Clock?"=FALSE) -> (w6879:T12)
                n3365 = property class="DigNum (strict)"(reference=w6878, "DisabledEnum"=T7."Enabled" ("Disabled")) -> ()  [unwired: 1 in, 2 out]
                n3366 = call "2pparameters.vi"("Params in"=w6879, "command"="set") -> ()  [unwired: 1 out]
              }
              frame True {
                n3367 = property class="DigNum (strict)"(reference=w6885, "Val(Sgnl)"=100000.0 ("Value (Signaling)"), "DisabledEnum"=T7."Disabled and Grayed Out" ("Disabled")) -> ()  [unwired: 1 in, 2 out]
                n3368 = call "2pparameters.vi"("command"="get") -> ("params out"=w6891:T12)  [unwired: 1 in]
                n3369 = Bundle By Name(cluster=w6891, "External 100KHz Clock?"=TRUE) -> (w6888:T12)
                n3370 = call "2pparameters.vi"("Params in"=w6888, "command"="set") -> ()  [unwired: 1 out]
              }
            }
          }
          event "Exit": Value Change {
            n3371 = event-data() -> ()  [unwired: 1 in, 5 out]
            n3372 = disable-structure shown="Enabled" {
              frame Disabled {
                # "added to see if it would fix crasing on exit"
                n3373 = call "ROI-databuffer.vi"("command"=enum16{"get", "set", "clear", "append"}."clear") -> ()  [unwired: 4 in, 1 out]
              }
              frame Enabled {
              }
            }
          }
        }
        n3374 = Wait (ms)(milliseconds to wait=u32 50) -> ()  [unwired: 1 out]
      }
      n3375 = while {
        stop <- w82 stop-if-true
        # "Waveform generation"
        n3376 = event shown="[21] \"Exit\": Value Change" {
          selector: _ -> [_ _ _ _ _ _ _ _ _ _ _ _ _ _ _ _ _ _ _ _ _ _]
          dyn-events: _ -> [_ _ _ _ _ _ _ _ _ _ _ _ _ _ _ _ _ _ _ _ _ _]
          timeout: _ -> [_ _ _ _ _ _ _ _ _ _ _ _ _ _ _ _ _ _ _ _ _ _]
          tunnel: [_ _ _ _ _ _ _ _ _ _ _ _ _ _ _ _ _ _ _ _ _ w2252] -> w82
          event Timeout {
            n3377 = event-data() -> ()  [unwired: 1 in, 3 out]
          }
          event "Add AO wave": Value Change {
            n3378 = event-data() -> ("NewVal"=w83:bool)  [unwired: 1 in, 5 out]
            n3379 = case shown="True" w83 {
              frame False {
              }
              frame True {
                n3380 = stacked-sequence {
                  seq-local: [_ _ w190 _ _ _ _ _] -> [_ _ _ w222 w233 w241 w307 w339]
                  frame #0 {
                    n3381 = local read "Measurement"() -> (w84:T4)
                    n3382 = case shown="\"Lifetime (contour)\"" w84 {
                      frame "X-Y-t movie", Default {
                        n3383 = local read "avpp"() -> (w105:i32)
                        n3384 = local read "Angle ref"() -> (w104:dbl)
                        n3385 = local read "ROI Type"() -> (w103:u16)
                        n3386 = local read "xpixels ref"() -> (w100:i32)
                        n3387 = local read "Vx-min ref"() -> (w99:dbl)
                        n3388 = local read "Vx-max ref"() -> (w98:dbl)
                        n3389 = local read "ypixels ref"() -> (w96:i32)
                        n3390 = local read "Vy-min ref"() -> (w97:dbl)
                        n3391 = local read "Vy-max ref"() -> (w93:dbl)
                        n3392 = local read "Sampling rate"() -> (w87:dbl)
                        n3393 = local read "finite samples"() -> (w88:bool)
                        n3394 = local read "continuous"() -> (w91:bool)
                        n3395 = local read "wavdet"() -> (w92:bool)
                        n3396 = local read "# of frames"() -> (w90:i32)
                        n3397 = local read "maxbufferAI"() -> (w89:i32)
                        n3398 = local read "Override AI buffer"() -> (w85:bool)
                        n3399 = call "2pparameters.vi"("command"="get") -> ("params out"=w102:T12)  [unwired: 1 in]
                        n3400 = Bundle By Name(cluster=w102, "type"="X-Y-t movie", "avpp"=w105, "Angle Img"=w104, "Xpixels Img"=w100, "Vx-min Img"=w99, "VX-max Img"=w98, "Ypixels Img"=w96, "Vy-min Img"=w97, "Vy-max Img"=w93, "srate"=w87, "srate Img"=w87, "finite"=w88, "cont"=w91, "wavdet"=w92, "measpoints"=w90, "maxbufferAI"=w89, "Drawing Mode"=w103, "Vz-reset"=0.0, "AIoverride"=w85) -> (w94:T12)
                        n3401 = call "2pparameters.vi"("Params in"=w94, "command"="set") -> ()  [unwired: 1 out]
                      }
                      frame "X-Y-Z stack" {
                        n3402 = call "2pparameters.vi"("command"="get") -> ("params out"=w109:T12)  [unwired: 1 in]
                        n3403 = Bundle By Name(cluster=w109, "type"="X-Y-Z stack") -> (w107:T12)
                        n3404 = call "2pparameters.vi"("Params in"=w107, "command"="set") -> ()  [unwired: 1 out]
                      }
                      frame "Lifetime (scan)" {
                        n3405 = call "2pparameters.vi"("command"="get") -> ("params out"=w114:T12)  [unwired: 1 in]
                        n3406 = Bundle By Name(cluster=w114, "type"="Lifetime (scan)") -> (w112:T12)
                        n3407 = call "2pparameters.vi"("Params in"=w112, "command"="set") -> ()  [unwired: 1 out]
                      }
                      frame "Lifetime (contour)" {
                        n3408 = local read "Vy-min draw"() -> (w124:dbl)
                        n3409 = local read "Vy-max draw"() -> (w123:dbl)
                        n3410 = local read "Vx-min draw"() -> (w126:dbl)
                        n3411 = local read "Vx-max draw"() -> (w125:dbl)
                        n3412 = local read "xpixels ref"() -> (w122:i32)
                        n3413 = local read "ypixels ref"() -> (w121:i32)
                        n3414 = local read "ROI Type"() -> (w120:u16)
                        n3415 = local read "srateAODOtt"() -> (w131:dbl)
                        n3416 = local read "# of frames"() -> (w136:i32)
                        n3417 = local read "refreshtime"() -> (w128:dbl)
                        n3418 = local read "Pel"() -> (w119:dbl)
                        n3419 = local read "bin"() -> (w134:dbl)
                        n3420 = local read "Override AI buffer"() -> (w117:bool)
                        n3421 = local read "finite samples"() -> (w143:bool)
                        n3422 = local read "srateAODOtt"() -> (w130:dbl)
                        n3423 = local read "srateAODOtt"() -> (w137:dbl)
                        n3424 = local read "continuous"() -> (w142:bool)
                        n3425 = local read "Angle ref"() -> (w127:dbl)
                        n3426 = local read "wavdet"() -> (w144:bool)
                        n3427 = local read "Vx-ref"() -> (w139:dbl)
                        n3428 = local read "Vy-ref"() -> (w141:dbl)
                        n3429 = local read "avpp"() -> (w140:i32)
                        n3430 = call "tt_timeandsamples.vi"("bin"=w134, "refreshtime"=w128, "srateAODOtt"=w131, "tot#ofsamples"=w136) -> ("refreshrate"=w132:dbl, "refreshbuffer"=w133:i32, "timetracecycles"=w138:i32)  [unwired: 5 in]
                        n3431 = local read "bin"() -> (w135:dbl)
                        n3432 = call "2pparameters.vi"("command"="get") -> ("params out"=w147:T12)  [unwired: 1 in]
                        n3433 = Bundle By Name(cluster=w147, "Drawing Mode"=w120, "measpoints"=w136, "tt_cycles"=w138, "refreshbuffer"=w133, "refreshrate"=w132, "Vx-ref"=w139, "Vy-ref"=w141, "srate"=w130, "finite"=w143, "cont"=w142, "wavdet"=w144, "avpp"=w140, "srateAODO"=w137, "bufferAI"=w133, "bin"=w135, "Angle Img"=w127, "Vxminref"=w126, "Vxmaxref"=w125, "Vyminref"=w124, "Vymaxref"=w123, "Xpixels Img"=w122, "Ypixels Img"=w121, "Pel"=w119, "Vz-reset"=0.0, "AIoverride"=w117, "type"="Lifetime (contour)") -> (w145:T12)
                        n3434 = Reciprocal(x=w132) -> (1/x=w129:dbl)
                        n3435 = local write "refreshtime"(w129) -> ()
                        n3436 = call "2pparameters.vi"("Params in"=w145, "command"="set") -> ()  [unwired: 1 out]
                      }
                      frame "X-Y-Z-t movie" {
                      }
                      frame "linescan" {
                      }
                      frame "Timetrace" {
                        n3437 = local read "Vy-min draw"() -> (w157:dbl)
                        n3438 = local read "Vy-max draw"() -> (w156:dbl)
                        n3439 = local read "Vx-min draw"() -> (w159:dbl)
                        n3440 = local read "Vx-max draw"() -> (w158:dbl)
                        n3441 = local read "xpixels ref"() -> (w155:i32)
                        n3442 = local read "ypixels ref"() -> (w154:i32)
                        n3443 = local read "ROI Type"() -> (w153:u16)
                        n3444 = local read "srateAODOtt"() -> (w164:dbl)
                        n3445 = local read "# of frames"() -> (w169:i32)
                        n3446 = local read "refreshtime"() -> (w161:dbl)
                        n3447 = local read "Pel"() -> (w152:dbl)
                        n3448 = local read "bin"() -> (w167:dbl)
                        n3449 = local read "Override AI buffer"() -> (w150:bool)
                        n3450 = local read "finite samples"() -> (w176:bool)
                        n3451 = local read "srateAODOtt"() -> (w163:dbl)
                        n3452 = local read "srateAODOtt"() -> (w170:dbl)
                        n3453 = local read "continuous"() -> (w175:bool)
                        n3454 = local read "Angle ref"() -> (w160:dbl)
                        n3455 = local read "wavdet"() -> (w177:bool)
                        n3456 = local read "Vx-ref"() -> (w172:dbl)
                        n3457 = local read "Vy-ref"() -> (w174:dbl)
                        n3458 = local read "avpp"() -> (w173:i32)
                        n3459 = call "tt_timeandsamples.vi"("bin"=w167, "refreshtime"=w161, "srateAODOtt"=w164, "tot#ofsamples"=w169) -> ("refreshrate"=w165:dbl, "refreshbuffer"=w166:i32, "timetracecycles"=w171:i32)  [unwired: 5 in]
                        n3460 = local read "bin"() -> (w168:dbl)
                        n3461 = call "2pparameters.vi"("command"="get") -> ("params out"=w180:T12)  [unwired: 1 in]
                        n3462 = Bundle By Name(cluster=w180, "Drawing Mode"=w153, "measpoints"=w169, "tt_cycles"=w171, "refreshbuffer"=w166, "refreshrate"=w165, "Vx-ref"=w172, "Vy-ref"=w174, "srate"=w163, "finite"=w176, "cont"=w175, "wavdet"=w177, "avpp"=w173, "srateAODO"=w170, "bufferAI"=w166, "bin"=w168, "Angle Img"=w160, "Vxminref"=w159, "Vxmaxref"=w158, "Vyminref"=w157, "Vymaxref"=w156, "Xpixels Img"=w155, "Ypixels Img"=w154, "Pel"=w152, "Vz-reset"=0.0, "AIoverride"=w150, "type"="Timetrace") -> (w178:T12)
                        n3463 = Reciprocal(x=w165) -> (1/x=w162:dbl)
                        n3464 = local write "refreshtime"(w162) -> ()
                        n3465 = call "2pparameters.vi"("Params in"=w178, "command"="set") -> ()  [unwired: 1 out]
                      }
                      frame "Lifetime (point)" {
                      }
                    }
                  }
                  frame #1 {
                    w183 = FALSE ("wavdet")
                    n3466 = call "2pparameters.vi"("command"="get") -> ("params out"=w187:T12)  [unwired: 1 in]
                    n3467 = Bundle By Name(cluster=w187, "finite"=w183, "cont"=w183, "wavdet"=TRUE) -> (w184:T12)
                    n3468 = call "2pparameters.vi"("Params in"=w184, "command"="set") -> ()  [unwired: 1 out]
                  }
                  frame #2 {
                    n3469 = local read "Meastab"() -> (w214:enum32{"X-Y Image", "Linescan", "Timetrace"})
                    n3470 = property on="AO channels" class="Ring (strict)"() -> ("RingText.Text"=w189:string)  [unwired: 2 in, 2 out]
                    n3471 = property on="refwf" class="Ring (strict)"() -> ("RingText.Text"=w213:string)  [unwired: 2 in, 2 out]
                    n3472 = local read "Build analog waveform tabs"() -> (w212:enum32{"Square", "Triangle", "Matlab"})
                    n3473 = case shown="\"X-Y Image\", Default" w214 {
                      tunnel: [w220 w221] -> w211
                      frame "X-Y Image", Default {
                        n3474 = local read "Sampling rate"() -> (w220:dbl)
                      }
                      frame "Timetrace" {
                        n3475 = local read "srateAODOtt"() -> (w221:dbl)
                      }
                    }
                    n3476 = local read "Matlab waveform path"() -> (w204:path)
                    n3477 = local read "Period (ms)"() -> (w207:dbl)
                    n3478 = local read "Frequency"() -> (w206:dbl)
                    n3479 = local read "Tri Repeats"() -> (w205:dbl)
                    n3480 = local read "Repeats"() -> (w210:dbl)
                    n3481 = local read "Cycles"() -> (w209:dbl)
                    n3482 = local read "Pulses"() -> (w208:dbl)
                    n3483 = call "matlabwfexistsdialogue.vi"("Matlab waveform path"=w204) -> ("mtalab waveform path out"=w203:path)
                    n3484 = call "wfsizecalc.vi"("Sampling frequency (Hz)"=w211, "AOtab"=w212, "reference waveforms to"=w213, "channel"=w189, "Repeats"=w210, "Cycles"=w209, "Matlab wave file"=w203, "pulses"=w208, "Period (ms)"=w207, "Frequency"=w206, "Tri Repeats"=w205) -> ("total size GB"=w198:dbl, "gigabytesize wf"=w194:dbl)  [unwired: 3 in]
                    n3485 = Greater?(x=w194, y=0.5) -> (0:w195:bool)
                    n3486 = Number To Fractional String(number=w194, width (-)=i16 3) -> (F-format string=w200:string)  [unwired: 2 in]
                    n3487 = Number To Fractional String(number=w198, width (-)=i16 4) -> (F-format string=w199:string)  [unwired: 2 in]
                    n3488 = Concatenate Strings("this is a crude approximation:\nyou're about to create a  " ("message"), w200, " GB waveform for a total of " ("string"), w199, " GB. Are you sure?" ("string")) -> (w196:string)
                    n3489 = case shown="True" w195 {
                      tunnel: w196 -> [_ w219]
                      tunnel: [TRUE ("T button?") w216] -> w190
                      frame False {
                      }
                      frame True {
                        n3490 = Two Button Dialog(message=w219, 1:"No, don't do this." ("Center Button Text (\"No\")"), 2:"Yes, continue. " ("Left Button Text (\"Yes\")")) -> (T button?=w216:bool)
                      }
                    }
                  }
                  frame #3 {
                    n3491 = case shown="True" w222 {
                      frame False {
                      }
                      frame True {
                        # "change active waveform numbers array"
                        n3492 = local read "AO channels"() -> (w228:u32)
                        n3493 = call "2pparameters.vi"("command"="get") -> ("params out"=w226:T12)  [unwired: 1 in]
                        n3494 = in-place {
                          in-place-border: w228 -> [w232]
                          in-place-border: [w229] -> w223
                          n3495 = in-place-cluster #48(w226) -> ("aAO"=w231:u32[])
                          n3496 = call "add channel to active arrayv2.vi"("line array in"=w231, "line to add"=w232) -> ("line array out"=w230:u32[], "addition"=w229:bool)  [unwired: 1 out]
                          n3497 = in-place-cluster #48("aAO"=w230) -> (w224:T12)
                        }
                        n3498 = local write "addAO"(w223) -> ()
                        n3499 = call "2pparameters.vi"("Params in"=w224, "command"="set") -> ()  [unwired: 1 out]
                      }
                    }
                  }
                  frame #4 {
                    n3500 = case shown="True" w233 {
                      frame False {
                      }
                      frame True {
                        # "update GUI"
                        n3501 = local read "addAO"() -> (w234:bool)
                        n3502 = case shown="True" w234 {
                          frame False {
                          }
                          frame True {
                            n3503 = call "Used AO lines.vi"() -> ("used AO names"=w238:string[], "used AO lines"=w240:tag[])  [unwired: 2 in]
                            n3504 = control-ref of="Analog Lines Plot"() -> (w239:refnum<vi>)
                            n3505 = control-ref of="Digital Lines Plot"() -> (w237:refnum<vi>)
                            n3506 = call "Used DO lines.vi"() -> ("used DO names"=w236:string[], "used DO lines"=w235:tag[])  [unwired: 2 in]
                            n3507 = local write "Analog Used Lines"(w240) -> ()
                            n3508 = local write "Analog Used Names"(w238) -> ()
                            n3509 = local write "Digital Used Lines"(w235) -> ()
                            n3510 = local write "Digital Used Names"(w236) -> ()
                            n3511 = call "prepDOWaveplot.vi"("DigitalGraph in"=w237, "used DO names"=w236) -> ()  [unwired: 1 in]
                            n3512 = call "prepAOWaveplot.vi"("WaveformGraph in"=w239, "Analog Used Names"=w238) -> ()  [unwired: 1 in]
                          }
                        }
                      }
                    }
                  }
                  frame #5 {
                    n3513 = case shown="True" w241 {
                      frame False {
                      }
                      frame True {
                        n3514 = local read "addAO"() -> (w242:bool)
                        n3515 = case shown="True" w242 {
                          frame False {
                          }
                          frame True {
                            # "add parameters\nto parameter array"
                            n3516 = local read "Build analog waveform tabs"() -> (w243:enum32{"Square", "Triangle", "Matlab"})
                            n3517 = case shown="\"Matlab\"" w243 {
                              frame "Square", Default {
                                w256 = 0.0 ("Offset (V)")
                                n3518 = local read "Meastab"() -> (w245:enum32{"X-Y Image", "Linescan", "Timetrace"})
                                n3519 = call "waveformparamsv2.vi"("command"="get") -> ("Params out"=w254:T17)  [unwired: 4 in, 2 out]
                                n3520 = Unbundle By Name(w254) -> ("AO parameters"=w251:T18)
                                n3521 = case shown="\"Timetrace\"" w245 {
                                tunnel: [w267 w268] -> w244
                                frame "X-Y Image", Default {
                                n3522 = local read "Sampling rate"() -> (w267:dbl)
                                }
                                frame "Timetrace" {
                                n3523 = local read "srateAODOtt"() -> (w268:dbl)
                                }
                                }
                                n3524 = local read "Start amplitude (V)"() -> (w264:dbl)
                                n3525 = local read "phase shift (ms)"() -> (w257:dbl)
                                n3526 = local read "Step size (V)"() -> (w262:dbl)
                                n3527 = local read "Baseline (V)"() -> (w263:dbl)
                                n3528 = local read "Period (ms)"() -> (w260:dbl)
                                n3529 = local read "padding value"() -> (w247:dbl)
                                n3530 = local read "Repeats"() -> (w266:dbl)
                                n3531 = local read "DC (%)"() -> (w261:dbl)
                                n3532 = local read "Cycles"() -> (w265:dbl)
                                n3533 = local read "Pulses"() -> (w258:dbl)
                                n3534 = Index Array(array=w251, index=0) -> (element=w252:T19)
                                n3535 = Bundle By Name(cluster=w252, "AOtab"=0.0 ("Repeats"), "Repeats"=w266, "Cycles"=w265, "Start amplitude (V)"=w264, "Baseline (V)"=w263, "Step size (V)"=w262, "DC (%)"=w261, "Sampling frequency (Hz)"=w244, "Period (ms)"=w260, "Offset (V)"=w256, "Amplitude (V)"=w256, "Frequency"=w256, "Tri Repeats"=w256, "phase shift (ms)"=w257, "Pulses"=w258, "Matlab wave file"=path "", "padding value"=w247) -> (w249:T19)
                                n3536 = Build Array(w249) -> (w248:T18)
